vi "Example Callback.vi"() -> ()   [LabVIEW 2010]
uses:
  C:/tf/play/labview/Tinkerforge.dll
  Tinkerforge.dll
panel:
  out "y (G)":sgl
  out "z (G)":sgl
  in  "stop":bool
  out "x (G)":sgl
  in  "uid":string="abc"
  in  "port":i32=4223
  in  "host":string="localhost"
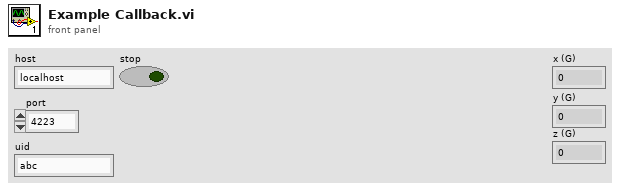
[diagram p1: front panel]
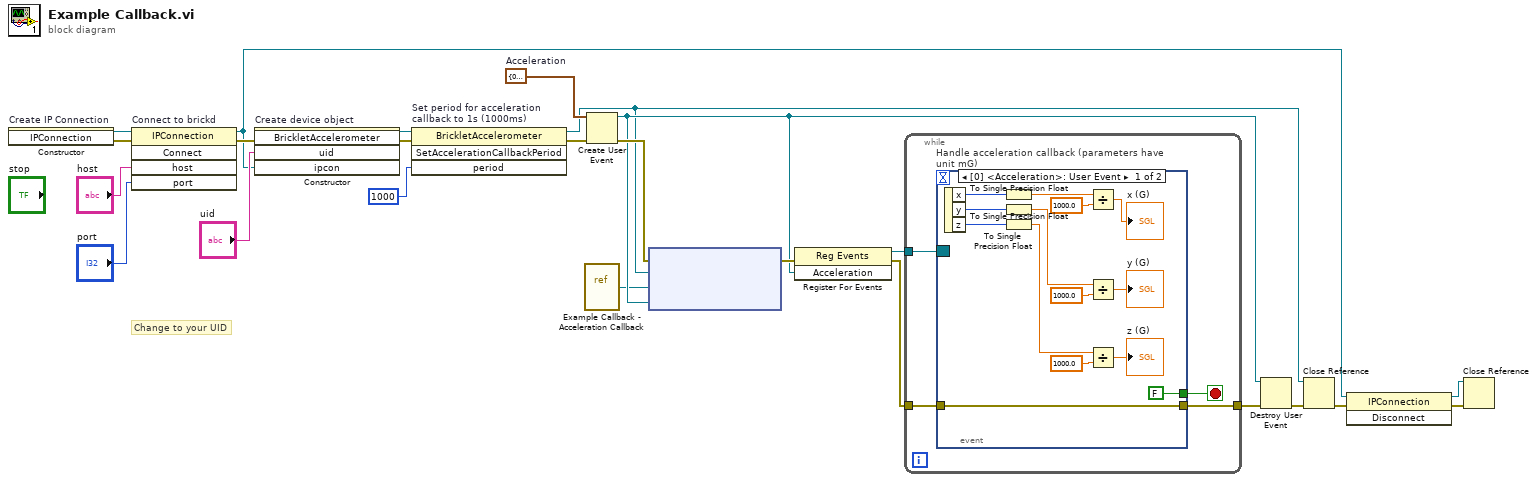
[diagram p0: block diagram]
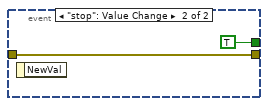
[diagram p2: hidden frame]
diagram:
  w8 = cluster{"x":i16, "y":i16, "z":i16} {"x"=0, "y"=0, "z"=0}  # Acceleration
  # "Change to your UID"
  n1 = constructor on="Create IP Connection" class="IPConnection"() -> (reference out=w24:refnum<k24>, error out=w2:errorcluster)  [unwired: 3 in, 1 out]
  n2 = invoke on="Connect to brickd" class="IPConnection" method="Connect"(reference=w24, error in=w2, "host"="host", "port"="port") -> (reference out=w17:refnum<k24>, error out=w20:errorcluster)  [unwired: 1 in, 3 out]
  n3 = constructor on="Create device object" class="BrickletAccelerometer"(error in=w20, "uid"="uid", "ipcon"=w17) -> (reference out=w5:refnum<k24>, error out=w7:errorcluster)  [unwired: 2 in, 3 out]
  n4 = invoke on="Set period for acceleration\ncallback to 1s (1000ms)" class="BrickletAccelerometer" method="SetAccelerationCallbackPeriod"(reference=w5, error in=w7, "period"=i64 1000) -> (reference out=w4:refnum<k24>, error out=w6:errorcluster)  [unwired: 1 in, 2 out]
  n5 = vi-ref "Example Callback - Acceleration Callback.vi"() -> ("vi reference"=w1:refnum<vi>)
  n6 = Create User Event(user event datatype=w8, error in=w6) -> (user event=w10:refnum<user-event>, error out=w15:errorcluster)
  n7 = node ("Register Event Callback")(w15, w4, w1, w10) -> (w14:errorcluster)  [unwired: 1 in, 1 out]
  n8 = register-events(error in=w14, w10) -> (reference out=w13:refnum<event-registration>, error out=w11:errorcluster)  [unwired: 1 in]
  n9 = while {
    tunnel: w13 -> [w28]
    tunnel: [w27] -> w12
    tunnel: w11 -> [w26]
    stop <- w25 stop-if-true
    n10 = event "Handle acceleration callback (parameters have unit mG)" shown="[0] <Acceleration>: User Event" {
      selector: w28 -> [_ _]
      dyn-events: _ -> [_ _]
      timeout: _ -> [_ _]
      tunnel: [w42 w43] -> w27
      tunnel: w26 -> [w42 w43]
      tunnel: [FALSE TRUE] -> w25
      event User Event {
        n11 = event-data() -> ("x"=w38:i16, "y"=w39:i16, "z"=w40:i16)  [unwired: 1 in]
        n12 = To Single Precision Float(number=w38) -> (single precision float=w37:sgl)
        n13 = To Single Precision Float(number=w39) -> (single precision float=w35:sgl)
        n14 = To Single Precision Float(number=w40) -> (single precision float=w33:sgl)
        n15 = Divide(x=w37, y=sgl 1000.0) -> (x/y=→"x (G)":sgl)
        n16 = Divide(x=w35, y=sgl 1000.0) -> (x/y=→"y (G)":sgl)
        n17 = Divide(x=w33, y=sgl 1000.0) -> (x/y=→"z (G)":sgl)
      }
      event "stop": Value Change {
        n18 = event-data() -> ()  [unwired: 1 in, 1 out]
      }
    }
  }
  n19 = Destroy User Event(user event=w10, error in=w12) -> (error out=w9:errorcluster)
  n20 = Close Reference(reference=w4, error in (no error)=w9) -> (error out=w19:errorcluster)
  n21 = invoke class="IPConnection" method="Disconnect"(reference=w17, error in=w19) -> (reference out=w16:refnum<k24>, error out=w18:errorcluster)  [unwired: 1 in, 1 out]
  n22 = Close Reference(reference=w16, error in (no error)=w18) -> ()  [unwired: 1 out]
